vi "Main.vi"() -> ()   [LabVIEW 2017]
doc: "This template is for the Queued Message Handler design pattern.\n\nThe Event Handling Loop generates messages based on user interface actions.\n\nThe Message Handling Loop processes messages generated by the Event Handling Loop, or by other messages. The messages are string values, so new messages can be added easily to the Message Cases case structure in the Message Handling Loop. Each message cluster can also provide an optional value for Message Data, which is a variant that can be converted to whatever message-specific data is required."
uses:
  <vilib>/Utility/config.llb/Config Data RefNum.ctl
  <instrlib>/Dynamixel XL320 (Drivers instrument)/Public/Motor Operation/Low Level/XL320_Baud Setting.ctl
  support/Message Queue/Enqueue Message (Single).vi
  <vilib>/Utility/error.llb/Error Cluster From Error Code.vi
  <vilib>/ErrorRing/Error Ring.xnode
  support/Message Queue/Message Queue.lvlib
  <vilib>/Utility/config.llb/NI_LVConfig.lvlib
  Desktop/Dynamixel XL320.lvlib
panel:
  in  "Random":bool
  in  "Emotion":i32(knob) scale=0.0..8.0
  in  "Stockage des indicateurs":enum32{"Fichier de config", "Motor"}(tab)
  out "Config.ini refnum":T1
  out "section names":string[](array[string])
  out "Nombre d'émotion":i32
  out "VISA resource name":refnum<visa-resource-name>
  in  "Exit":bool
  # "Contact : Ghislain REMY\nGhislain.remy@u-psud.fr"
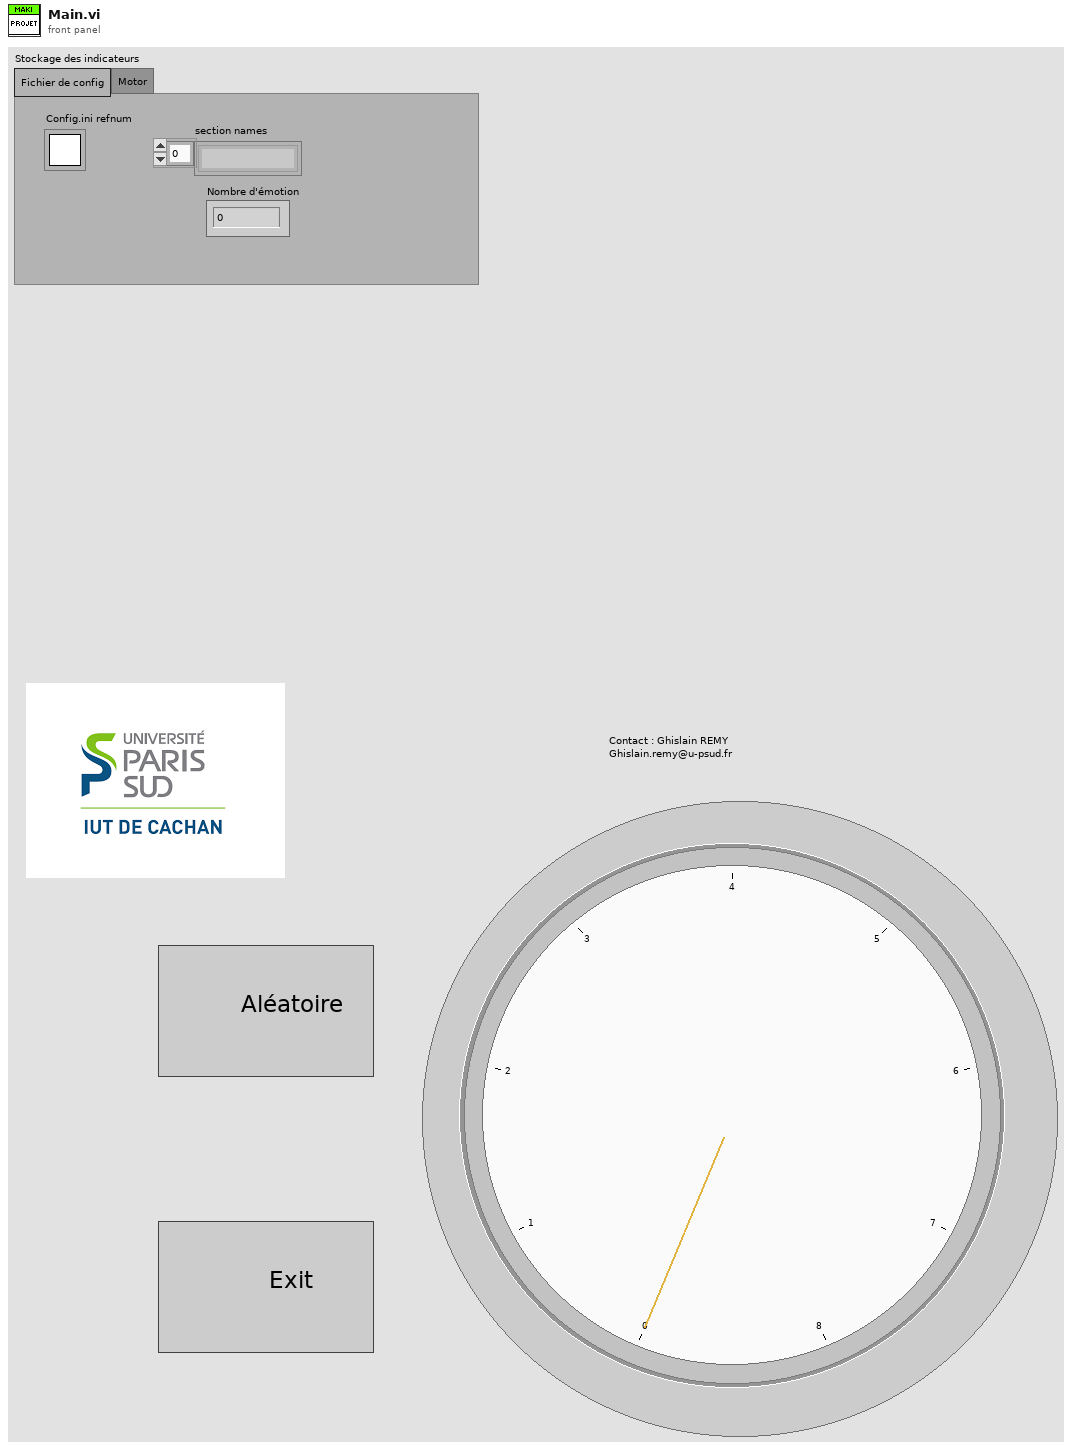
[diagram p1: front panel]
types:
  T1 = typedef "NI_LVConfig.lvlib/Config Data RefNum.ctl" = refnum<k1>
  T2 = typedef "Message Queue.lvlib/All Message Queues.ctl" = cluster{"UI":refnum<queue>}
  T3 = typedef "Dynamixel XL320.lvlib/XL320_Baud Setting.ctl" = u8
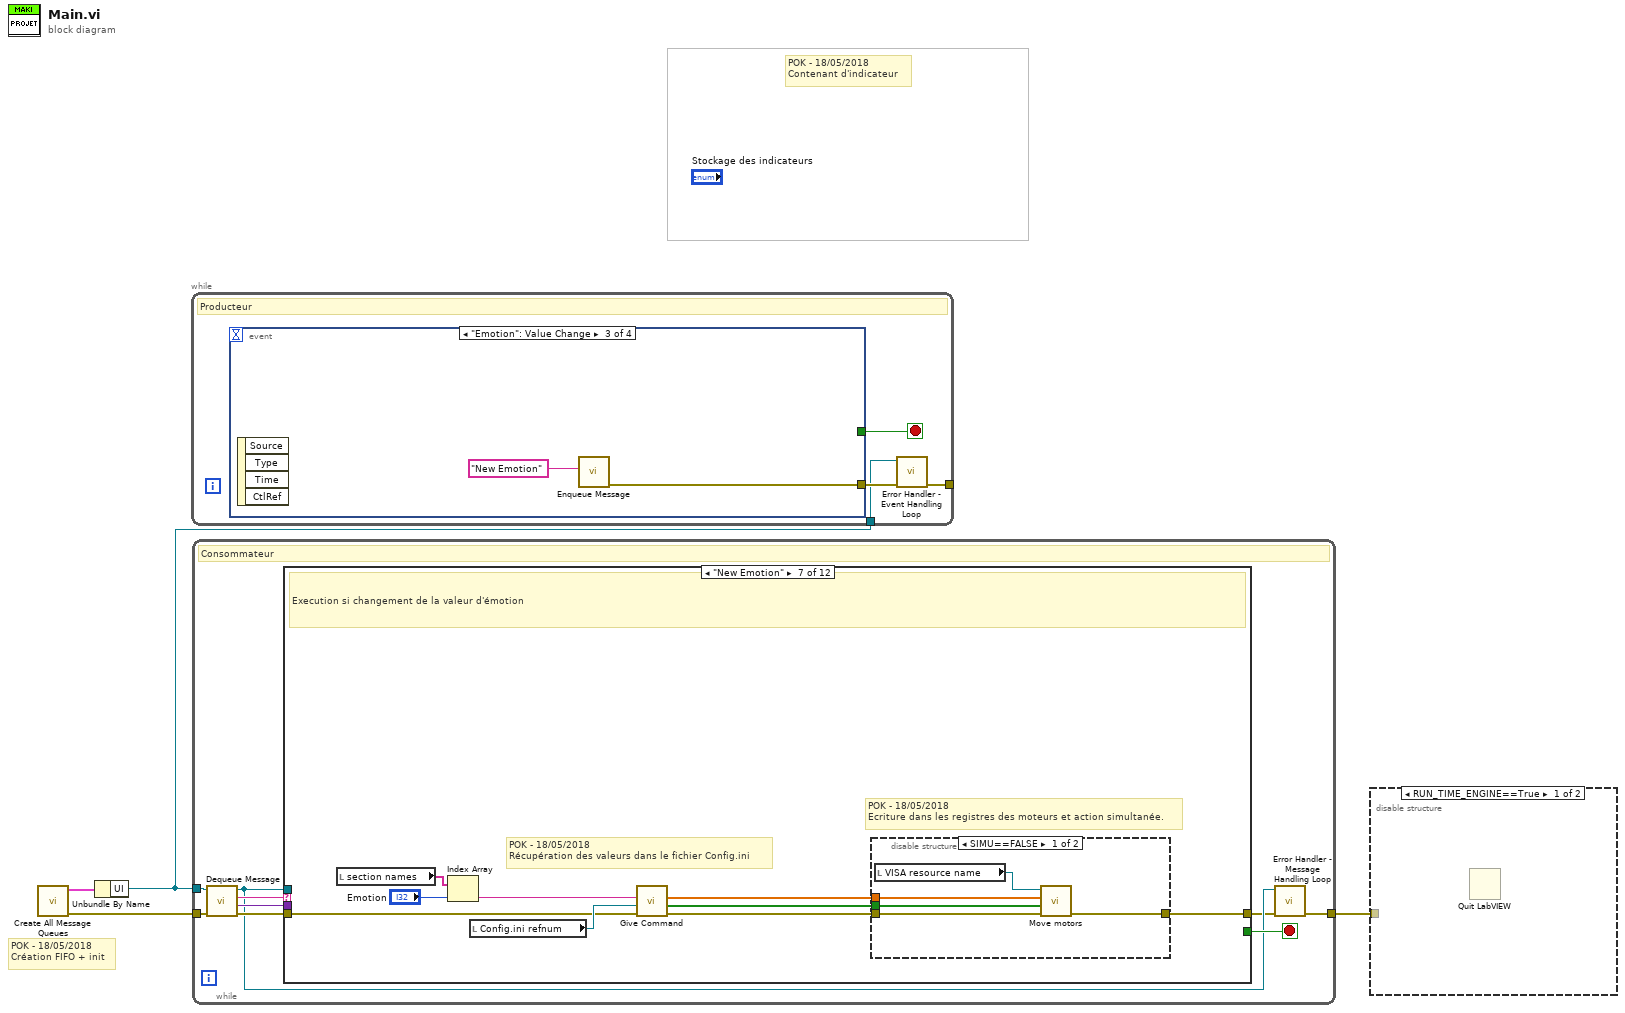
[diagram p0: block diagram]
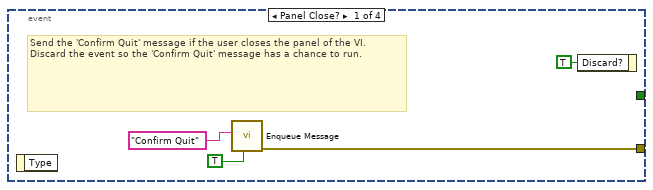
[diagram p3: hidden frame]
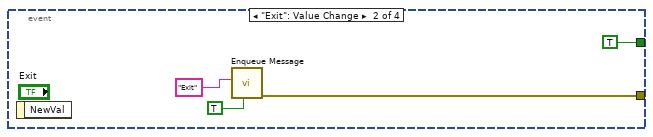
[diagram p4: hidden frame]
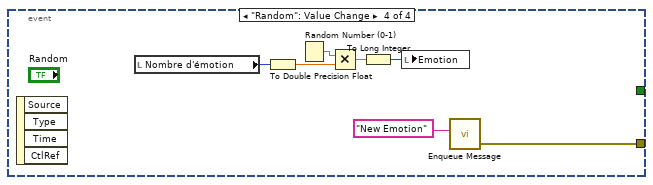
[diagram p5: hidden frame]
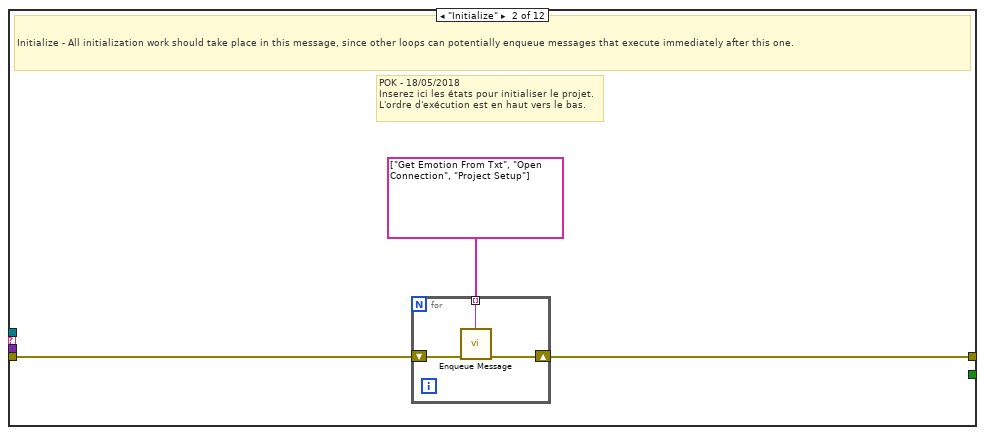
[diagram p7: hidden frame]
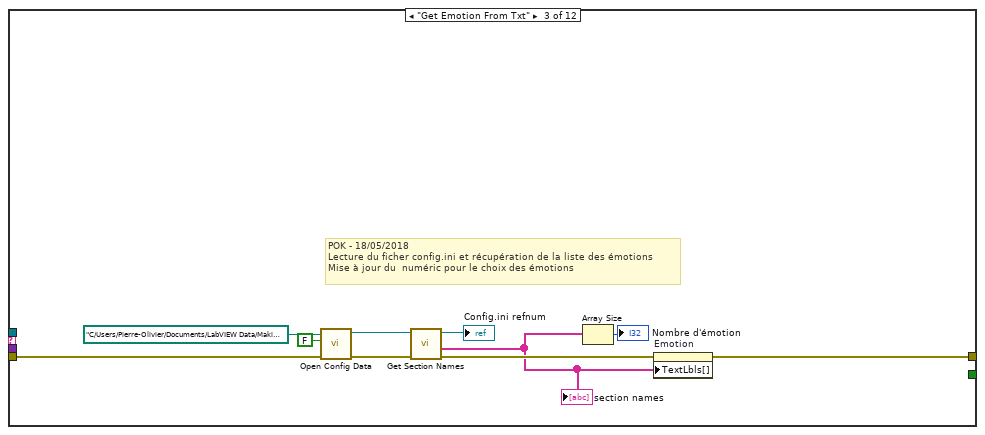
[diagram p8: hidden frame]
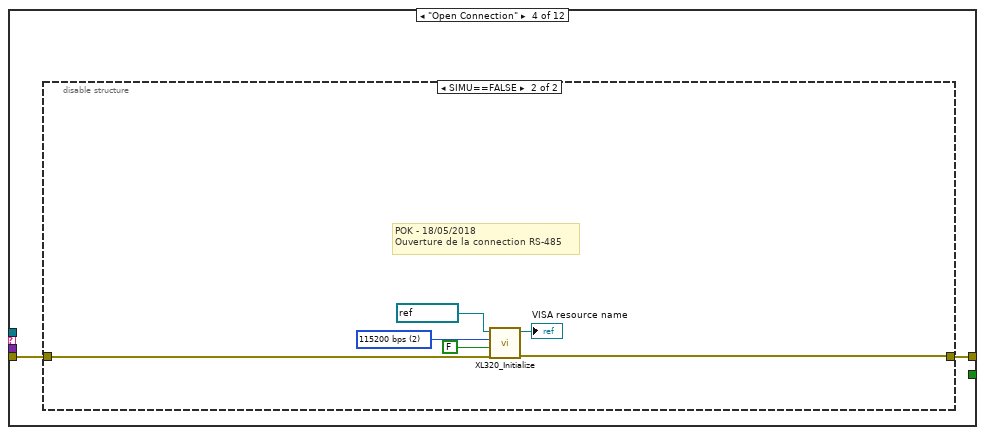
[diagram p9: hidden frame]
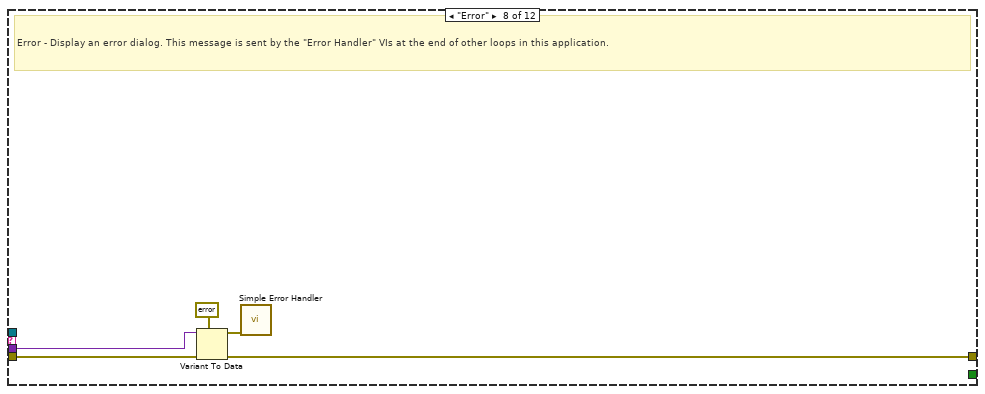
[diagram p14: hidden frame]
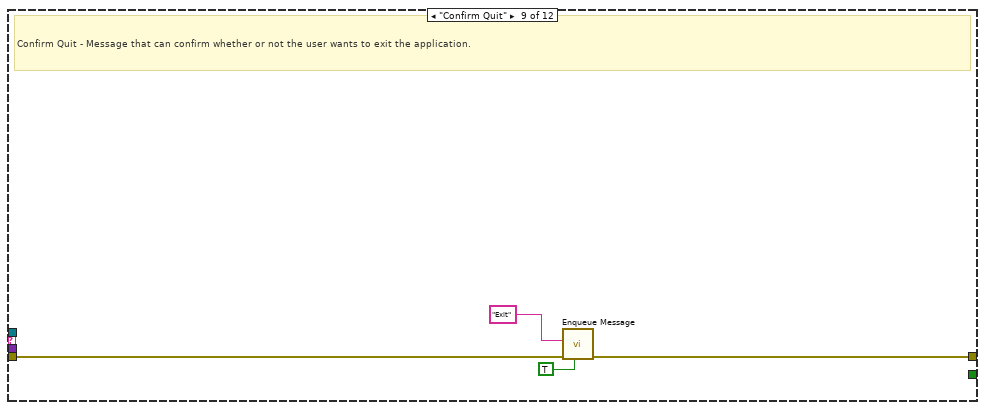
[diagram p15: hidden frame]
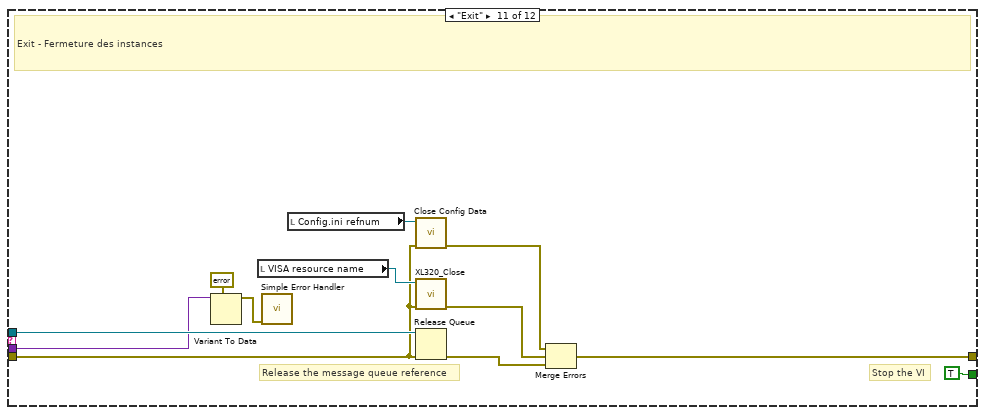
[diagram p17: hidden frame]
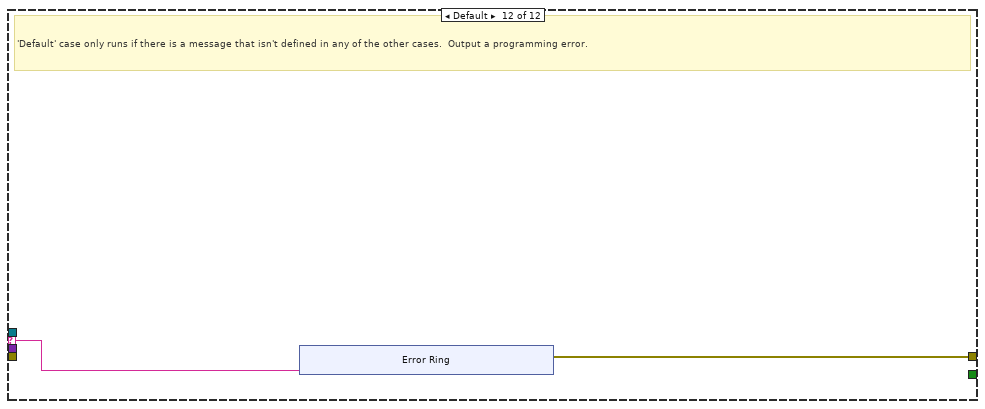
[diagram p18: hidden frame]
diagram:
  # "POK - 18/05/2018\nContenant d'indicateur"
  # "POK - 18/05/2018\nCréation FIFO + init"
  n1 = call "Create All Message Queues.vi"() -> ("error out"=w4:errorcluster, "Message Queues out"=w3:T2)  [unwired: 10 in]
  n2 = Unbundle By Name(w3) -> ("UI"=w2:refnum<queue>)
  n3 = while {
    tunnel: [w6] -> _
    tunnel: w2 -> [w5]
    stop <- w7 stop-if-true
    # "Producteur"
    n4 = event shown="[2] \"Emotion\": Value Change" {
      selector: _ -> [_ _ _ _]
      dyn-events: _ -> [_ _ _ _]
      timeout: _ -> [_ _ _ _]
      tunnel: [_ TRUE _ _] -> w7
      tunnel: [w11 w16 w17 w19] -> w8
      event Panel Close? {
        # "Send the 'Confirm Quit' message if the user closes the panel of the VI. Discard the event so the 'Confirm Quit' message has a chance to run."
        n5 = event-data() -> ()  [unwired: 1 in, 1 out]
        n6 = call-poly "Enqueue Message.vi"("Priority Message? (F)"=TRUE, "Message"="Confirm Quit") -> ("error out"=w11:errorcluster)  [unwired: 8 in, 1 out]
        n7 = event-data("Discard?"=TRUE) -> ()  [unwired: 1 in, 1 out]
      }
      event "Exit": Value Change {
        n8 = event-data() -> ()  [unwired: 1 in, 1 out]
        n9 = call-poly "Enqueue Message.vi"("Priority Message? (F)"=TRUE, "Message"="Exit") -> ("error out"=w16:errorcluster)  [unwired: 8 in, 1 out]
      }
      event "Emotion": Value Change {
        n10 = event-data() -> ()  [unwired: 1 in, 4 out]
        n11 = call-poly "Enqueue Message.vi"("Message"="New Emotion") -> ("error out"=w17:errorcluster)  [unwired: 9 in, 1 out]
      }
      event "Random": Value Change {
        n12 = event-data() -> ()  [unwired: 1 in, 4 out]
        n13 = local read "Nombre d'émotion"() -> (w25:i32)
        n14 = To Double Precision Float(number=w25) -> (double precision float=w24:dbl)
        n15 = Random Number (0-1)() -> (number: 0 to 1=w23:dbl)
        n16 = Multiply(x=w23, y=w24) -> (x*y=w22:dbl)
        n17 = To Long Integer(number=w22) -> (32bit integer=w21:i32)
        n18 = local write "Emotion"(w21) -> ()
        n19 = call-poly "Enqueue Message.vi"("Message"="New Emotion") -> ("error out"=w19:errorcluster)  [unwired: 9 in, 1 out]
      }
    }
    n20 = call "Error Handler - Event Handling Loop.vi"("error in (no error)"=w8, "Message Queue"=w5) -> ("dup error in"=w6:errorcluster)  [unwired: 8 in, 1 out]
  }
  n21 = while {
    tunnel: w2 -> [w29]
    tunnel: w4 -> [w33]
    tunnel: [w27] -> w1
    stop <- w34 stop-if-true
    # "Consommateur"
    n22 = call "Dequeue Message.vi"("error in (no error)"=w33, "Message Queue"=w29) -> ("error out"=w32:errorcluster, "Message Data"=w30:variant, "Message"=w31:string, "dup Message Queue"=w28:refnum<queue>)  [unwired: 6 in]
    n23 = case "Message Cases" shown="\"New Emotion\"" w31 {
      selector: w31 -> [_ _ _ _ _ _ _ _ _ _ _ w100]
      tunnel: w28 -> [_ _ _ _ _ _ _ _ _ _ w99 _]
      tunnel: w32 -> [w35 w38 w50 w52 w61 w62 w64 w82 w86 w87 w88 _]
      tunnel: [w35 w37 w44 w53 w61 w62 w67 w78 w85 w87 w97 w101] -> w26
      tunnel: [_ _ _ _ _ _ _ _ _ _ TRUE _] -> w34
      tunnel: w30 -> [_ _ _ _ _ _ _ w81 _ _ w94 _]
      frame "----- INITIALIZE ----" {
      }
      frame "Initialize" {
        # "POK - 18/05/2018\nInserez ici les états pour initialiser le projet.\nL'ordre d'exécution est en haut vers le bas."
        # "Initialize - All initialization work should take place in this message, since other loops can potentially enqueue messages that execute immediately after this one."
        n24 = for {
          shift-right: [w40] -> w37
          shift-left: w38 -> [w41]
          tunnel: string[] ["Get Emotion From Txt", "Open Connection", "Project Setup"] -> [w39] mode=indexing
          n25 = call-poly "Enqueue Message.vi"("error in (no error)"=w41, "Message"=w39) -> ("error out"=w40:errorcluster)  [unwired: 8 in, 1 out]
        }
      }
      frame "Get Emotion From Txt" {
        # "POK - 18/05/2018\nLecture du ficher config.ini et récupération de la liste des émotions\nMise à jour du  numéric pour le choix des émotions"
        n26 = call <vilib>:"Open Config Data.vi"("error in (no error)"=w50, "create file if necessary (T)"=FALSE, "configuration file path"=path "C:/Users/Pierre-Olivier/Documents/LabVIEW Data/Maki Project/Support Files/Configuration.ini") -> ("error out"=w51:errorcluster, "refnum"=w49:T1)  [unwired: 6 in, 1 out]
        n27 = call <vilib>:"Get Section Names.vi"("error in (no error)"=w51, "refnum"=w49) -> ("error out"=w45:errorcluster, "section names"=w43:string[], "refnum out"=→"Config.ini refnum":T1)  [unwired: 7 in]
        "section names" <- w43
        n28 = Array Size(array=w43) -> (size(s)=→"Nombre d'émotion":i32)
        n29 = property on="Emotion" class="Knob (strict)"(error in=w45, "TextLbls[]"=w43) -> (error out=w44:errorcluster)  [unwired: 1 in, 1 out]
      }
      frame "Open Connection" {
        n30 = disable-structure shown="SIMU==FALSE" {
          disable-tunnel: [w54 w59] -> w53
          disable-tunnel: w52 -> [w54 w60]
          frame condition #0 {
          }
          frame condition #1 (active) {
            w56 = T3 2 items=["9600 bps", "57600 bps", "115200 bps", "1,000,000 bps"] ("Baud rate (1,000,000 bps)")
            # "POK - 18/05/2018\nOuverture de la connection RS-485"
            n31 = call <instrlib>:"XL320_Initialize.vi"("error in (no error)"=w60, "Force Baud Rate (True)"=FALSE, "Baud rate (1,000,000 bps)"=w56, "VISA resource name"=refnum<visa-resource-name> "COM6") -> ("error out"=w59:errorcluster, "VISA resource name out"=→"VISA resource name":refnum<visa-resource-name>)  [unwired: 6 in]
          }
        }
      }
      frame "Project Setup" {
      }
      frame "-----PROJECT EXEC----" {
      }
      frame "New Emotion" {
        # "POK - 18/05/2018\nEcriture dans les registres des moteurs et action simultanée."
        # "POK - 18/05/2018\nRécupération des valeurs dans le fichier Config.ini"
        # "Execution si changement de la valeur d'émotion"
        n32 = local read "section names"() -> (w71:string[])
        n33 = Index Array(array=w71, index="Emotion") -> (element=w70:string)
        n34 = local read "Config.ini refnum"() -> (w69:T1)
        n35 = call "Give Command.vi"("Error In"=w64, "Config.ini refnum"=w69, "Emotion"=w70) -> ("Error Out"=w68:errorcluster, "Boolean_Array"=w65:bool[], "DBL_Array"=w66:dbl[])  [unwired: 6 in]
        n36 = disable-structure shown="SIMU==FALSE" {
          disable-tunnel: w68 -> [w76 w77]
          disable-tunnel: [w75 w77] -> w67
          disable-tunnel: w66 -> [w74 _]
          disable-tunnel: w65 -> [w73 _]
          frame condition #0 (active) {
            n37 = local read "VISA resource name"() -> (w72:refnum<visa-resource-name>)
            n38 = call "Move motors.vi"("Error In"=w76, "Boolean_Array"=w73, "Numeric_Array"=w74, "VISA resource name"=w72) -> ("Error Out"=w75:errorcluster)  [unwired: 7 in]
          }
          frame condition #1 {
          }
        }
      }
      frame "Error" {
        # "Error - Display an error dialog. This message is sent by the \"Error Handler\" VIs at the end of other loops in this application."
        n39 = Variant To Data(error in=w82, type=errorcluster {"status"=FALSE, "code"=0, "source"=""} ("error constant"), Variant=w81) -> (data=w79:errorcluster, error out=w78:errorcluster)
        n40 = call <vilib>:"Simple Error Handler.vi"("error in (no error)"=w79) -> ()  [unwired: 4 in, 5 out]
      }
      frame "Confirm Quit" {
        # "Confirm Quit - Message that can confirm whether or not the user wants to exit the application."
        n41 = call-poly "Enqueue Message.vi"("Priority Message? (F)"=TRUE, "error in (no error)"=w86, "Message"="Exit") -> ("error out"=w85:errorcluster)  [unwired: 7 in, 1 out]
      }
      frame "---Copy This Frame---" {
        # "Duplicate this frame when creating new messages.  Change this comment in the duplicated frame to describe this message."
      }
      frame "Exit" {
        # "Stop the VI"
        # "Release the message queue reference"
        # "Exit - Fermeture des instances"
        n42 = Variant To Data(type=errorcluster {"status"=FALSE, "code"=0, "source"=""} ("error constant"), Variant=w94) -> (data=w95:errorcluster)  [unwired: 1 in, 1 out]
        n43 = local read "VISA resource name"() -> (w89:refnum<visa-resource-name>)
        n44 = call <vilib>:"Simple Error Handler.vi"("error in (no error)"=w95) -> ()  [unwired: 4 in, 5 out]
        n45 = local read "Config.ini refnum"() -> (w92:T1)
        n46 = call <vilib>:"Close Config Data.vi"("error in (no error)"=w88, "refnum"=w92) -> ("error out"=w93:errorcluster)  [unwired: 8 in, 1 out]
        n47 = call <instrlib>:"XL320_Close.vi"("error in (no error)"=w88, "VISA resource name"=w89) -> ("error out"=w90:errorcluster)  [unwired: 9 in]
        n48 = Release Queue(queue=w99, error in (no error)=w88) -> (error out=w91:errorcluster)  [unwired: 1 in, 2 out]
        n49 = Merge Errors(w93, w90, w91) -> (w97:errorcluster)
      }
      frame Default {
        # "'Default' case only runs if there is a message that isn't defined in any of the other cases.  Output a programming error."
        n50 = xnode "Error Ring"("parameter 0"=w100) -> ("error out"=w101:errorcluster)
      }
    }
    n51 = call "Error Handler - Message Handling Loop.vi"("error in (no error)"=w26, "Message Queue"=w28) -> ("dup error in"=w27:errorcluster)  [unwired: 8 in, 1 out]
  }
  n52 = disable-structure shown="RUN_TIME_ENGINE==True" {
    disable-tunnel: w1 -> [_ _]
    frame condition #0 {
      n53 = Quit LabVIEW() -> ()  [unwired: 1 in]
    }
    frame condition #1 (active) {
    }
  }
